vi "GetRTC.vi"(8 "error in (no error)":errorcluster, 11 "reference in":refnum<class "Flux_Capacitor.lvclass">) -> (0 "error out":errorcluster, 1 "OK":bool, 2 "RTC":timestamp, 3 "reference in":refnum<class "Flux_Capacitor.lvclass">)   [LabVIEW 2022 SP3, in "Flux_Capacitor.lvlib" / "Flux_Capacitor.lvclass"]
uses:
  Flux_Capacitor.lvclass
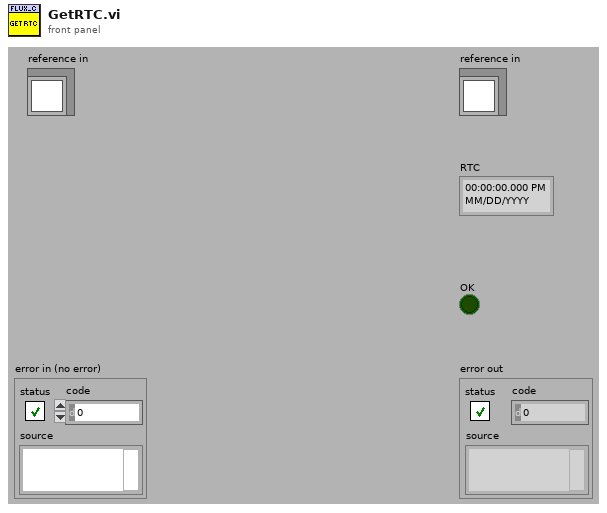
[diagram p1: front panel]
types:
  T1 = typedef "Flux_Capacitor.lvlib/Flux_Capacitor.lvclass/ObjectAttributes.ctl" = cluster{"Config":T2, "T Sensors":T3[], "Temp_DegC":dbl[], "Temp_Raw":u64[], "RTC":timestamp, "Flux":bool, "Time":timestamp, "RTC_Live":timestamp}
  T2 = typedef "Flux_Capacitor.lvlib/Flux_Capacitor.lvclass/Config.ctl" = cluster{"default":string}
  T3 = typedef "Flux_Capacitor.lvlib/Flux_Capacitor.lvclass/TempSensor.ctl" = enum16{"1", "2", "3"}
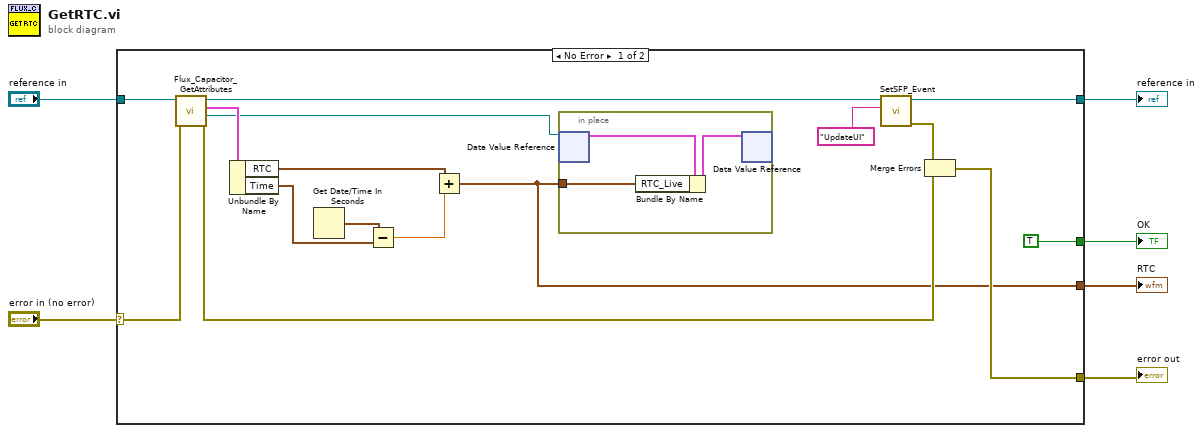
[diagram p0: block diagram]
diagram:
  n1 = case shown="No Error" "error in (no error)" {
    selector: "error in (no error)" -> [w22 w27]
    tunnel: [w16 w27] -> w5
    tunnel: [w15 w26] -> w3
    tunnel: "reference in" -> [w21 w26]
    tunnel: [TRUE _] -> w2
    tunnel: [w7 _] -> w1
    frame No Error {
      n2 = call "Flux_Capacitor_GetAttributes.vi"("error in (no error)"=w22, "reference in"=w21) -> ("error out"=w18:errorcluster, "DataRef"=w8:refnum<data-value>, "Data"=w14:T1, "reference out"=w17:refnum<class "Flux_Capacitor.lvclass">)  [unwired: 6 in]
      n3 = Unbundle By Name(w14) -> ("RTC"=w12:timestamp, "Time"=w9:timestamp)
      n4 = Get Date/Time In Seconds() -> (seconds since 1Jan1904=w10:timestamp)
      n5 = Subtract(x=w10, y=w9) -> (x-y=w13:dbl)
      n6 = Add(x=w12, y=w13) -> (x+y=w7:timestamp)
      n7 = in-place {
        in-place-border: w7 -> [w23]
        n8 = in-place-dvr #1(w8) -> (w25:T1)  [unwired: 1 out]
        n9 = Bundle By Name(cluster=w25, "RTC_Live"=w23) -> (w24:T1)
        n10 = in-place-dvr #1(w24) -> ()  [unwired: 2 out]
      }
      n11 = call-dynamic "SetSFP_Event.vi"("msg"="UpdateUI", "reference in"=w17) -> ("error out"=w20:errorcluster, "reference out"=w15:refnum<class "Flux_Capacitor.lvclass">)  [unwired: 8 in]
      n12 = Merge Errors(w20, w18) -> (w16:errorcluster)
    }
    frame Error {
    }
  }
  "error out" <- w5
  "reference in" <- w3
  "OK" <- w2
  "RTC" <- w1
